vi "próbnik.vi"(11 "output cluster 2":T1) -> (3 "Message Cluster":T2, 7 "number stopy":u32)   [LabVIEW 2015]
uses:
  QMH Fundamentals - Message Cluster.ctl
  CANFrameControl.ctl
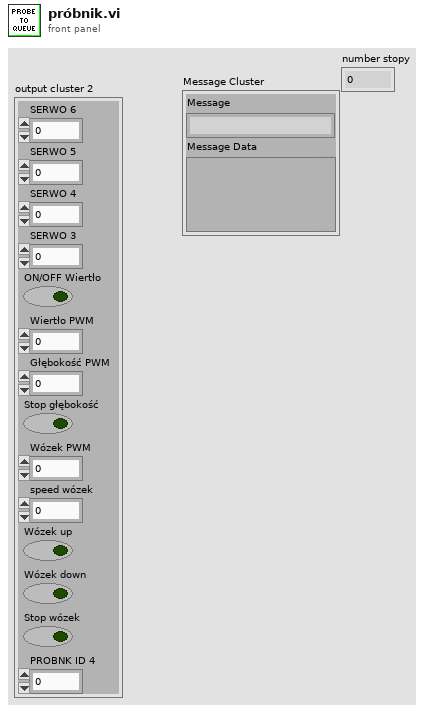
[diagram p1: front panel]
types:
  T1 = cluster{"SERWO 6":u8, "SERWO 5":u8, "SERWO 4":u8, "SERWO 3":u8, "ON/OFF Wiertło":bool, "Wiertło PWM":u8, "Głębokość PWM":u8, "Stop głębokość":bool, "Wózek PWM":u8, "speed wózek":u8, "Wózek up":bool, "Wózek down":bool, "Stop wózek":bool, "PROBNK ID 4":u32}
  T2 = typedef "QMH Fundamentals - Message Cluster.ctl" = cluster{"Message":string, "Message Data":variant}
  T3 = typedef "CANFrameControl.ctl" = cluster{"identifier":u32, "extended?":bool, "type":u8, "payload":u8[]}
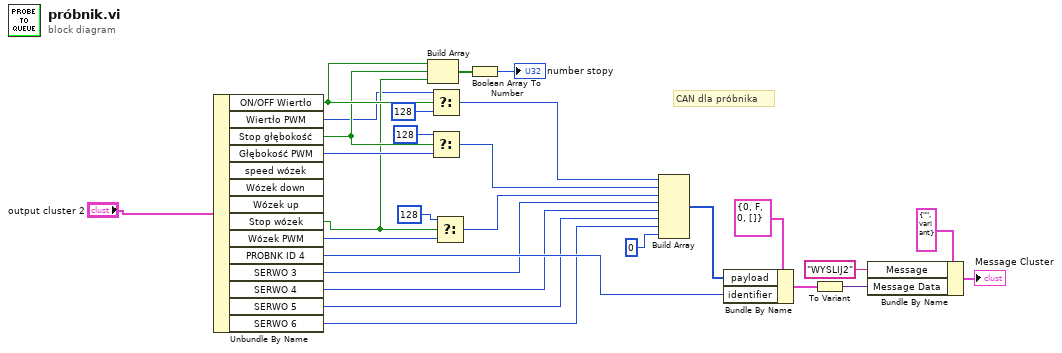
[diagram p0: block diagram]
diagram:
  # "CAN dla próbnika"
  n1 = Unbundle By Name("output cluster 2") -> ("ON/OFF Wiertło"=w13:bool, "Wiertło PWM"=w7:u8, "Stop głębokość"=w12:bool, "Głębokość PWM"=w16:u8, "Stop wózek"=w11:bool, "Wózek PWM"=w19:u8, "PROBNK ID 4"=w21:u32, "SERWO 3"=w6:u8, "SERWO 4"=w3:u8, "SERWO 5"=w2:u8, "SERWO 6"=w1:u8)  [unwired: 3 out]
  n2 = Build Array(w13, w12, w11) -> (w10:bool[])
  n3 = Select(t=w7, s=w13, f=u8 128) -> (s? t:f=w15:u8)
  n4 = Select(t=u8 128, s=w12, f=w16) -> (s? t:f=w14:u8)
  n5 = Select(t=u8 128, s=w11, f=w19) -> (s? t:f=w18:u8)
  n6 = Boolean Array To Number(Boolean array=w10) -> (number=→"number stopy":u32)
  n7 = Build Array(w15, w14, w18, w6, w3, w2, w1, u8 0) -> (w22:u8[])
  n8 = Bundle By Name(cluster=T3 {"identifier"=0, "extended?"=FALSE, "type"=0, "payload"=[]} ("CAN frame 2"), "payload"=w22, "identifier"=w21) -> (w28:T3)
  n9 = To Variant(anything=w28) -> (Variant=w24:variant)
  n10 = Bundle By Name(cluster=T2 {"Message"="", "Message Data"=variant} ("Message Cluster"), "Message"="WYSLIJ2", "Message Data"=w24) -> (→"Message Cluster":T2)
